vi "64x128OLED_SSD1315_Graph.vi"() -> ()   [LabVIEW 2024]
uses:
  Driver/Public/Digital Pull Direction.ctl
  <vilib>/picture/cartesn2.llb/XY Plot Type.ctl
  a7562c57-8a3f-42dc-a248-a218528d61d2.vi
  6f0d1129-d4e0-4dc5-a4b8-79dcd5bf0572.vi
  Public/GetPicture.vi
  Public/BuildMessagesFromPicture.vi
  Public/InitialiseOLED.vi
  Driver/CTIPicoVISA.lvlib
  OLEDI2CMessageGenerator.lvlib
panel:
  out "Numeric":i32
  in  "stop":bool
  out "2D Picture":picture
  in  "Grove Connector":enum16{"I2C0", "I2C1"}(ring)
  out "Identity":T1
  out "error out":errorcluster={"status"=TRUE, "code"=15, "source"="CTI.lvlib:Session.lvclass:Check I2C Pins.vi:4130001<ERR>\nInvalid pin selection for I2C:\nGPIO 5 is invalid for I2C 1 SCL, valid options: 3, 7, 11, 15, 19, 27\r\nGPIO 4 is invalid for I2C 1 SDA, valid options: 2, 6, 10, 14, 18, 26\n\n\n<b>Complete call chain:</b>\r\n     CTI.lvlib:Session.lvclass:Check I2C Pins.vi:4130001\r\n     CTI.lvlib:Session.lvclass:Reserve I2C.vi\r\n     CTI.lvlib:Session.lvclass:Configure I2C.vi:7080001\r\n     I2CLCD1602.vi"}
  in  "Port":refnum<visa-resource-name>="COM7"
  # "https://wiki.seeedstudio.com/Grove-OLED-Display-0.96-SSD1315/"
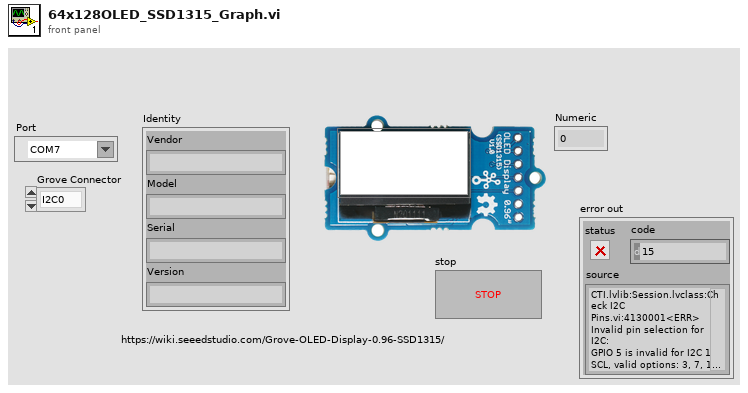
[diagram p1: front panel]
types:
  T1 = cluster{"Vendor":string, "Model":string, "Serial":string, "Version":string}
  T2 = cluster{"Font Name:":string, "Size":i16, "Strikeout?":bool, "Italic?":bool, "Underline?":bool, "Outline?":bool, "Shadow?":bool, "Bold?":bool}
  T3 = typedef "CTIPicoVISA.lvlib/Digital Pull Direction.ctl" = enum16{"None", "Up", "Down", "Both"}
  T4 = cluster{"line color":u32, "text color":u32, "tick length(3)":i16, "crossing axes":bool, "visible grid?":bool}
  T5 = typedef "XY Plot Type.ctl" = enum16{"points", "squares", "circles", "connected points", "connected squares", "connected circles", "comb plot", "sized scatter plot", "sized-colored scatter plot", "min-max lines"}
  T6 = cluster{"plot color":u32, "XY plot type":T5, "baseline":dbl}
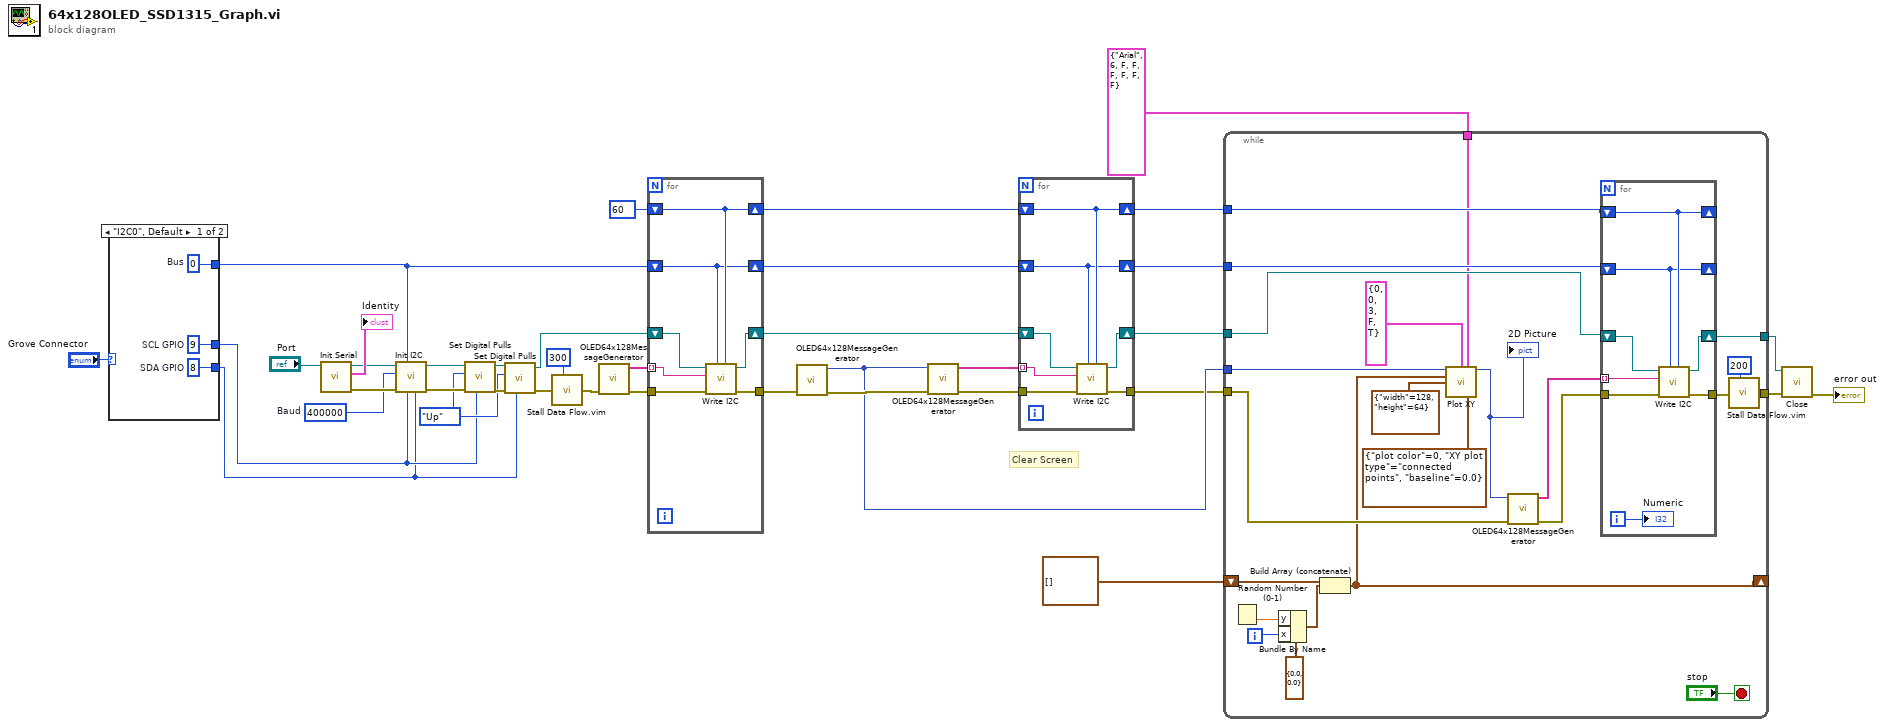
[diagram p0: block diagram]
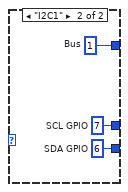
[diagram p2: hidden frame]
diagram:
  w29 = Digital_Pull_Direction."Up" ("Pull")
  w24 = u32 400000  # Baud
  # "Clear Screen"
  n1 = case shown="\"I2C0\", Default" "Grove Connector" {
    tunnel: [w41 w44] -> w17
    tunnel: [w40 w43] -> w16
    tunnel: [w39 w42] -> w22
    frame "I2C0", Default {
      w39 = u8 0  # Bus
      w40 = 8  # SDA GPIO
      w41 = 9  # SCL GPIO
    }
    frame "I2C1" {
      w42 = u8 1  # Bus
      w43 = 6  # SDA GPIO
      w44 = 7  # SCL GPIO
    }
  }
  n2 = call "Init Serial.vi"("VISA resource name in"="Port") -> ("error out"=w25:errorcluster, "Identity"=→"Identity":T1, "VISA resource name Out"=w26:refnum<visa-resource-name>)  [unwired: 8 in]
  n3 = call "Init I2C.vi"("SDA GPIO"=w16, "SCL GPIO"=w17, "Bus"=w22, "error in (no error)"=w25, "Baud"=w24, "VISA resource name in"=w26) -> ("error out"=w32:errorcluster, "VISA resource name"=w33:refnum<visa-resource-name>)  [unwired: 4 in]
  n4 = call "Set Digital Pulls.vi"("GPIO"=w17, "error in (no error)"=w32, "Pull"=w29, "VISA resource name in"=w33) -> ("error out"=w30:errorcluster, "VISA resource name"=w31:refnum<visa-resource-name>)  [unwired: 6 in]
  n5 = call "Set Digital Pulls.vi"("GPIO"=w16, "error in (no error)"=w30, "Pull"=w29, "VISA resource name in"=w31) -> ("error out"=w13:errorcluster, "VISA resource name"=w12:refnum<visa-resource-name>)  [unwired: 6 in]
  n6 = call "Stall Data Flow.vim"("value in"=w13, "milliseconds to wait"=u32 300) -> ("value out"=w27:errorcluster)  [unwired: 1 out]
  n7 = call-poly "OLED64x128MessageGenerator.vi"("error in (no error)"=w27) -> ("error out"=w23:errorcluster, "Messages"=w34:string[])  [unwired: 9 in]
  n8 = for {
    tunnel: w34 -> [w49] mode=indexing
    tunnel: w23 -> [w51]
    tunnel: [w48] -> w20
    shift-right: [w47] -> w7
    shift-left: w12 -> [w50]
    shift-right: [w46] -> w8
    shift-left: u8 60 ("Address") -> [w46]
    shift-right: [w45] -> w6
    shift-left: w22 -> [w45]
    n9 = call "Write I2C.vi"("Address"=w46, "Bus"=w45, "error in (no error)"=w51, "Data"=w49, "VISA resource name in"=w50) -> ("error out"=w48:errorcluster, "VISA resource name"=w47:refnum<visa-resource-name>)  [unwired: 5 in]
  }
  n10 = call-poly "OLED64x128MessageGenerator.vi"("error in (no error)"=w20) -> ("error out"=w15:errorcluster, "2D Picture"=w14:picture)  [unwired: 9 in]
  n11 = call-poly "OLED64x128MessageGenerator.vi"("error in (no error)"=w15, "2D Picture"=w14) -> ("error out"=w11:errorcluster, "Messages"=w10:string[])  [unwired: 8 in]
  n12 = for {
    tunnel: w10 -> [w56] mode=indexing
    tunnel: w11 -> [w58]
    tunnel: [w55] -> w9
    shift-right: [w54] -> w5
    shift-left: w7 -> [w57]
    shift-right: [w53] -> w3
    shift-left: w8 -> [w53]
    shift-right: [w52] -> w4
    shift-left: w6 -> [w52]
    n13 = call "Write I2C.vi"("Address"=w53, "Bus"=w52, "error in (no error)"=w58, "Data"=w56, "VISA resource name in"=w57) -> ("error out"=w55:errorcluster, "VISA resource name"=w54:refnum<visa-resource-name>)  [unwired: 5 in]
  }
  n14 = while {
    tunnel: w14 -> [w69]
    tunnel: w9 -> [w81]
    tunnel: w3 -> [w80]
    tunnel: w4 -> [w79]
    tunnel: w5 -> [w78]
    tunnel: [w75] -> w18
    tunnel: [w72] -> w19
    tunnel: T2 {"Font Name:"="Arial", "Size"=6, "Strikeout?"=FALSE, "Italic?"=FALSE, "Underline?"=FALSE, "Outline?"=FALSE, "Shadow?"=FALSE, "Bold?"=FALSE} ("[user-specified font]") -> [w67]
    shift-right: [w61] -> _
    shift-left: cluster{"x":dbl, "y":dbl}[] [] ("data") -> [w63]
    i -> [w65]
    stop <- "stop" stop-if-true
    n15 = Random Number (0-1)() -> (number: 0 to 1=w64:dbl)
    n16 = Bundle By Name(cluster=cluster{"x":dbl, "y":dbl} {"x"=0.0, "y"=0.0} ("Point [horizontal, vertical]"), "y"=w64, "x"=w65) -> (w62:cluster{"x":dbl, "y":dbl})
    n17 = Build Array (concatenate)(w63, w62) -> (w61:cluster{"x":dbl, "y":dbl}[])
    n18 = call <vilib>:"Plot XY.vi"("picture"=w69, "[user-specified font]"=w67, "data"=w61, "dimensions (w,h)"=cluster{"width":i16, "height":i16} {"width"=128, "height"=64}, "cartesian grid cosmetics"=T4 {"line color"=0, "text color"=0, "tick length(3)"=3, "crossing axes"=FALSE, "visible grid?"=TRUE}, "XY plot cosmetics"=T6 {"plot color"=0, "XY plot type"=enum."connected points", "baseline"=0.0}) -> ("new picture"=w70:picture)  [unwired: 9 in]
    "2D Picture" <- w70
    n19 = call-poly "OLED64x128MessageGenerator.vi"("error in (no error)"=w81, "2D Picture"=w70) -> ("error out"=w77:errorcluster, "Messages"=w76:string[])  [unwired: 8 in]
    n20 = for {
      tunnel: w76 -> [w87] mode=indexing
      tunnel: w77 -> [w89]
      tunnel: [w86] -> w73
      shift-right: [w85] -> w75
      shift-left: w78 -> [w88]
      shift-right: [w84] -> _
      shift-left: w80 -> [w84]
      shift-right: [w83] -> _
      shift-left: w79 -> [w83]
      i -> [w82]
      n21 = call "Write I2C.vi"("Address"=w84, "Bus"=w83, "error in (no error)"=w89, "Data"=w87, "VISA resource name in"=w88) -> ("error out"=w86:errorcluster, "VISA resource name"=w85:refnum<visa-resource-name>)  [unwired: 5 in]
      "Numeric" <- w82
    }
    n22 = call "Stall Data Flow.vim"("value in"=w73, "milliseconds to wait"=u32 200) -> ("value out"=w72:errorcluster)  [unwired: 1 out]
  }
  n23 = call "Close.vi"("error in (no error)"=w19, "VISA resource name in"=w18) -> ("error out"=→"error out":errorcluster)  [unwired: 9 in]
